vi "ExSubOpenInitCamera.vi"(0 "error in (no error)":errorcluster) -> (1 "Camera Handle":u32, 2 "error out":errorcluster)   [LabVIEW 2010]
uses:
  GlobalCamHandle.vi
  GlobalCamOpen.vi
  GlobalCCDMaxDim.vi
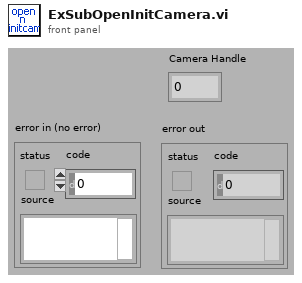
[diagram p1: front panel]
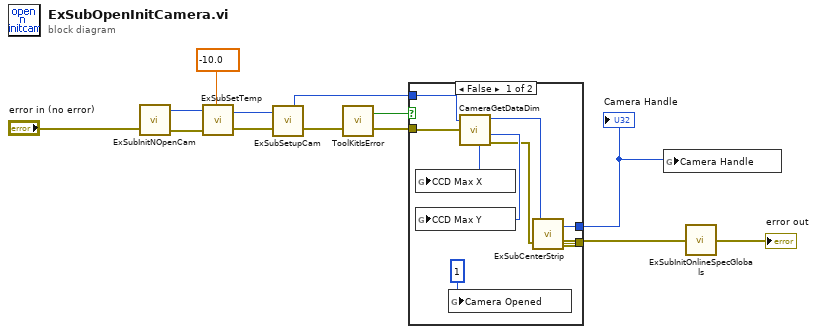
[diagram p0: block diagram]
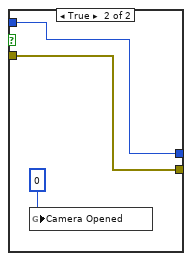
[diagram p2: hidden frame]
diagram:
  n1 = call "ExSubInitNOpenCam.vi"("error in (no error)"="error in (no error)") -> ("Camera Handle"=w11:u32, "error out"=w12:errorcluster)
  n2 = call "ExSubSetTemp.vi"("error in (no error)"=w12, "Temperature"=-10.0, "CameraHandle"=w11) -> ("error out"=w9:errorcluster, "Camera Handle"=w8:u32)
  n3 = call "ExSubSetupCam.vi"("error in (no error)"=w9, "Camera Handle"=w8) -> ("error out"=w5:errorcluster, "Camera Handle"=w4:u32)
  n4 = call <userlib>:"ToolKitIsError.vi"("error in"=w5) -> ("error out"=w6:errorcluster, "Error Flag"=w7:bool)  [unwired: 1 in]
  n5 = case shown="False" w7 {
    tunnel: w6 -> [w21 w23]
    tunnel: w4 -> [w16 w24]
    tunnel: [w15 w24] -> w3
    tunnel: [w14 w23] -> w2
    frame False {
      n6 = global write "GlobalCamOpen.vi" "Camera Opened"(1) -> ()
      n7 = call <userlib>:"CameraGetDataDim.vi"("Camera Handle"=w16, "error in"=w21) -> ("Camera Handle"=w18:u32, "Xdim"=w20:u32, "Ydim"=w19:u32, "error out"=w17:errorcluster)
      n8 = global write "GlobalCCDMaxDim.vi" "CCD Max X"(w20) -> ()
      n9 = global write "GlobalCCDMaxDim.vi" "CCD Max Y"(w19) -> ()
      n10 = call "ExSubCenterStrip.vi"("error in (no error)"=w17, "Camera Handle"=w18) -> ("error out"=w14:errorcluster, "Camera Handle"=w15:u32)
    }
    frame True {
      n11 = global write "GlobalCamOpen.vi" "Camera Opened"(0) -> ()
    }
  }
  "Camera Handle" <- w3
  n12 = global write "GlobalCamHandle.vi" "Camera Handle"(w3) -> ()
  n13 = call "ExSubInitOnlineSpecGlobals.vi"("error in (no error)"=w2) -> ("error out"=→"error out":errorcluster)
